vi "Rotation Matrix to Angle Vector.vi"(0 "rotation matrix":T1) -> (1 "angle":dbl, 2 "vector":dbl[](array[numeric]))   [LabVIEW 2021]
doc: "This VI transforms rotation matrix to angle vector."
uses:
  <vilib>/Analysis/Matrix/Datatypes/RealMatrix.ctl
  <vilib>/Analysis/_algsub.llb/Real Matrix Trace.vi
  <vilib>/Analysis/_algsub.llb/Real Vector Norm.vi
  <vilib>/Analysis/NI_AALPro.lvlib
  <vilib>/Analysis/Matrix/NI_Matrix.lvlib
panel:
  # "This VI transforms rotation matrix to angle vector."
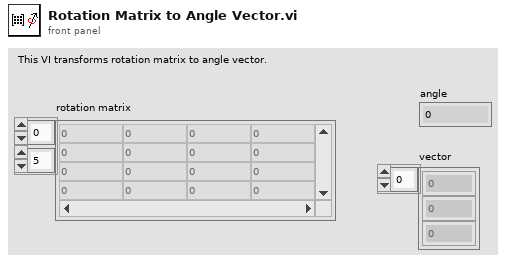
[diagram p1: front panel]
types:
  T1 = typedef "NI_Matrix.lvlib/RealMatrix.ctl" = dbl[][]
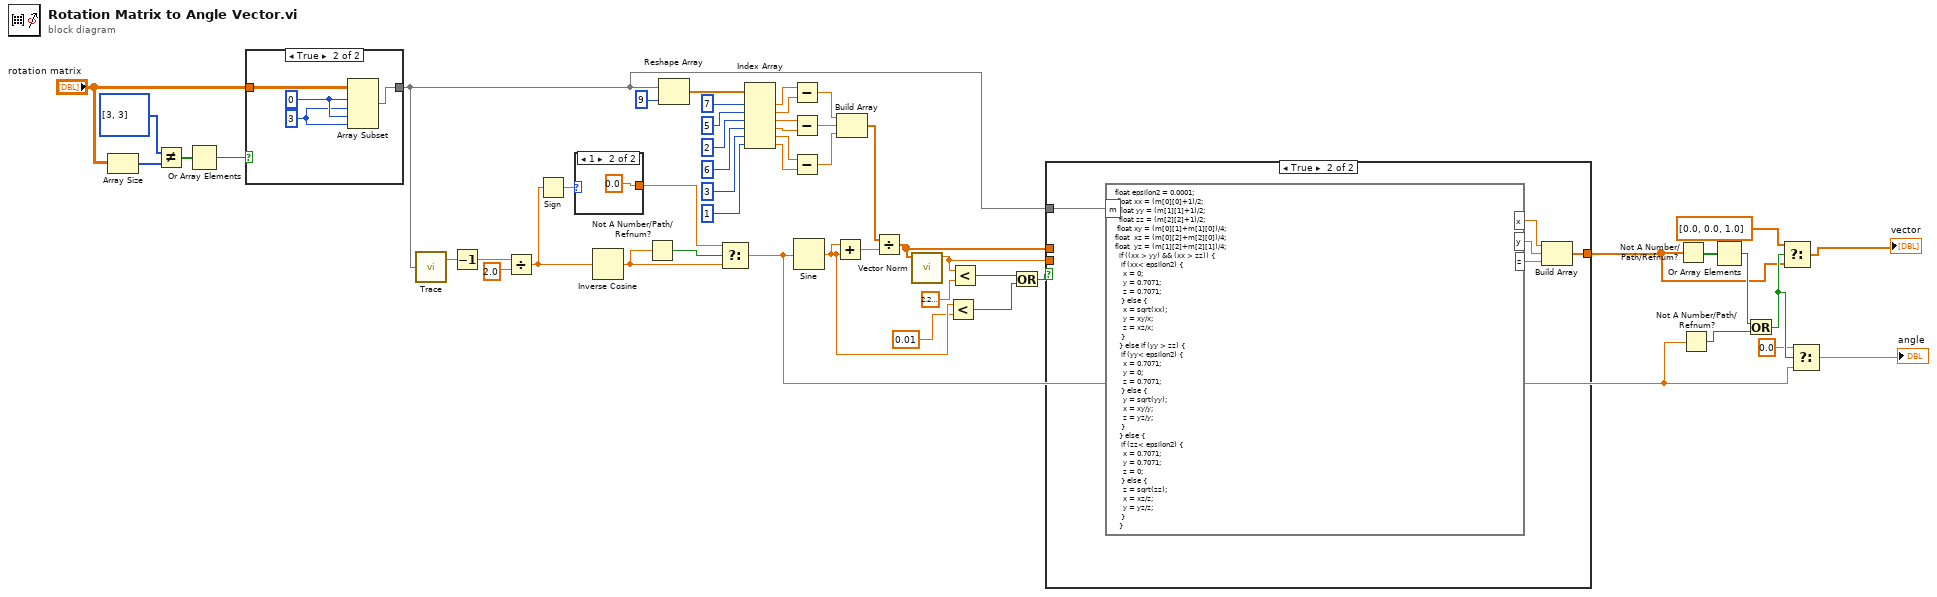
[diagram p0: block diagram]
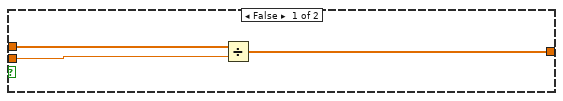
[diagram p2: hidden frame]
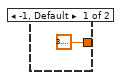
[diagram p3: hidden frame]
diagram:
  n1 = Array Size(array="rotation matrix") -> (size(s)=w51:i32[])
  n2 = Not Equal?(x=i32[] [3, 3] ("y"), y=w51) -> (x != y?=w49:bool[])
  n3 = Or Array Elements(Boolean array=w49) -> (logical OR=w48:bool)
  n4 = case shown="True" w48 {
    tunnel: [w52 w53] -> w19
    tunnel: "rotation matrix" -> [w52 w54]
    frame False {
    }
    frame True {
      w55 = 3 ("length")
      w56 = 0 ("index")
      n5 = Array Subset(array=w54, index (row)=w56, length (row)=w55, index (col)=w56, length (col)=w55) -> (w53:T1)
    }
  }
  n6 = call-poly <vilib>:"Trace.vi"("Input Matrix"=w19) -> ("trace"=w45:dbl)  [unwired: 1 out]
  n7 = Decrement(x=w45) -> (x-1=w46:dbl)
  n8 = Divide(x=w46, y=2.0) -> (x/y=w44:dbl)
  n9 = Sign(1:w44) -> (0:w43:dbl)
  n10 = case shown="1" w43 {
    tunnel: [3.141592653589793 0.0] -> w41
    frame -1, Default {
    }
    frame 1 {
    }
  }
  n11 = Inverse Cosine(1:w44) -> (0:w40:dbl)
  n12 = Not A Number/Path/Refnum?(number/path/refnum=w40) -> (NaN/Path/Refnum?=w42:bool)
  n13 = Reshape Array(w19, 9 ("dimension size")) -> (w20:dbl[])
  n14 = Select(t=w41, s=w42, f=w40) -> (s? t:f=w2:dbl)
  n15 = Index Array(array=w20, index #1=7 ("index"), index #2=5 ("index"), index #3=2 ("index"), index #4=6 ("index"), index #5=3 ("index"), index #6=1 ("index")) -> (element #1=w32:dbl, element #2=w33:dbl, element #3=w29:dbl, element #4=w28:dbl, element #5=w31:dbl, element #6=w30:dbl)
  n16 = Subtract(x=w32, y=w33) -> (x-y=w27:dbl)
  n17 = Subtract(x=w29, y=w28) -> (x-y=w26:dbl)
  n18 = Subtract(x=w31, y=w30) -> (x-y=w25:dbl)
  n19 = Sine(x=w2) -> (sin(x)=w15:dbl)
  n20 = Add(x=w15, y=w15) -> (x+y=w24:dbl)
  n21 = Build Array(w27, w26, w25) -> (w23:dbl[])
  n22 = Divide(x=w23, y=w24) -> (x/y=w21:dbl[])
  n23 = call-poly <vilib>:"Vector Norm.vi"("Input Vector"=w21) -> ("norm"=w18:dbl)  [unwired: 9 in, 1 out]
  n24 = Less?(x=w15, y=0.01) -> (x < y?=w13:bool)
  n25 = Less?(x=w18, y=2.220446049250313e-16) -> (x < y?=w16:bool)
  n26 = Or(x=w16, y=w13) -> (x .or. y?=w12:bool)
  n27 = case shown="True" w12 {
    tunnel: w21 -> [w61 _]
    tunnel: w18 -> [w60 _]
    tunnel: [w59 w62] -> w5
    tunnel: w19 -> [_ w66]
    frame False {
      n28 = Divide(x=w61, y=w60) -> (x/y=w59:dbl[])
    }
    frame True {
      n29 = formula code="float epsilon2 = 0.0001;  \n float xx = (m[0][0]+1)/2;\n\t\tfloat yy = (m[1][1]+1)/2;\n\t\tfloat zz = (m[2][2]+1)/2;\n\tfloat\txy = (m[0][1]+m[1][0])/4;\nfloat\t\txz = (m[0][2]+m[2][0])/4;\nfloat\t\tyz = (m[1][2]+m[2][1])/4;\n\t\tif ((xx > yy) && (xx > zz)) { \n\t\t\tif (xx< epsilon2) {\n\t\t\t\tx = 0;\n\t\t\t\ty = 0.7071;\n\t\t\t\tz = 0.7071;\n\t\t\t} else {\n\t\t\t\tx = sqrt(xx);\n\t\t\t\ty = xy/x;\n\t\t\t\tz = xz/x;\n\t\t\t}\n\t\t} else if (yy > zz) {\n\t\t\tif (yy< epsilon2) {\n\t\t\t\tx = 0.7071;\n\t\t\t\ty = 0;\n\t\t\t\tz = 0.7071;\n\t\t\t} else {\n\t\t\t\ty = sqrt(yy);\n\t\t\t\tx = xy/y;\n\t\t\t\tz = yz/y;\n\t\t\t}\t\n\t\t} else {\n\t\t\tif (zz< epsilon2) {\n\t\t\t\tx = 0.7071;\n\t\t\t\ty = 0.7071;\n\t\t\t\tz = 0;\n\t\t\t} else {\n\t\t\t\tz = sqrt(zz);\n\t\t\t\tx = xz/z;\n\t\t\t\ty = yz/z;\n\t\t\t}\n\t\t}"("m"=w66) -> ("x"=w65:dbl, "y"=w64:dbl, "z"=w63:dbl)
      n30 = Build Array(w65, w64, w63) -> (w62:dbl[])
    }
  }
  n31 = Not A Number/Path/Refnum?(number/path/refnum=w5) -> (NaN/Path/Refnum?=w11:bool[])
  n32 = Not A Number/Path/Refnum?(number/path/refnum=w2) -> (NaN/Path/Refnum?=w8:bool)
  n33 = Or Array Elements(Boolean array=w11) -> (logical OR=w9:bool)
  n34 = Or(x=w9, y=w8) -> (x .or. y?=w7:bool)
  n35 = Select(t=dbl[] [0.0, 0.0, 1.0], s=w7, f=w5) -> (s? t:f=→"vector":dbl[])
  n36 = Select(t=0.0, s=w7, f=w2) -> (s? t:f=→"angle":dbl)
